vi "final drive.vi"() -> ()   [LabVIEW 2012, in "Sendmail.lvrbt"]
uses:
  Sendmail.lvrbt
  <vilib>/NXT/Block Support/NXT_MessageMailbox.ctl
  <vilib>/NXT/Hardware/Plugins/Tetrix 180 deg Servo/Tetrix180ServoAddress.ctl
  <vilib>/NXT/Hardware/Plugins/Tetrix DC Motor/TetrixDCMotorAddress.ctl
  <vilib>/NXT/Dual Mode Library/BT/BlueTooth_Read_string.vi
  <vilib>/NXT/NXTIO Xnodes/NXTIONodeSubVIs/TETRIX IO Move Servos.vi
  <vilib>/NXT/Dual Mode Library/Display/drawNumber_float.vi
  <vilib>/NXT/Dual Mode Library/Display/drawText.vi
  <vilib>/NXT/NXTIO Xnodes/NXTIONodeSubVIs/TETRIX IO Move DC Motors.vi
  <vilib>/NXT/Subs/LVHSConnector.ctl
  <vilib>/NXT/NXTIO Xnodes/AddressXNode/NXTIOAddress.xnode
  <vilib>/NXT/NXTIO Xnodes/NXTIOXNode/NXTIO.xnode
  <vilib>/NXT/LegoClasses/BrickReference/BrickReference.lvclass
panel:
  in  "String":string
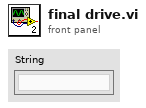
[diagram p1: front panel]
types:
  T1 = typedef "TetrixDCMotorAddress.ctl" = i16
  T2 = cluster{"TetrixDCMotor":T1, "TetrixDCMotor 2":T1}
  T3 = typedef "Tetrix180ServoAddress.ctl" = i16
  T4 = cluster{"Tetrix180Servo":T3, "Tetrix180Servo 2":T3}
  T5 = typedef "NXT_MessageMailbox.ctl" = u8
  T6 = cluster{"Tetrix180Servo":T3, "Tetrix180Servo":T3}
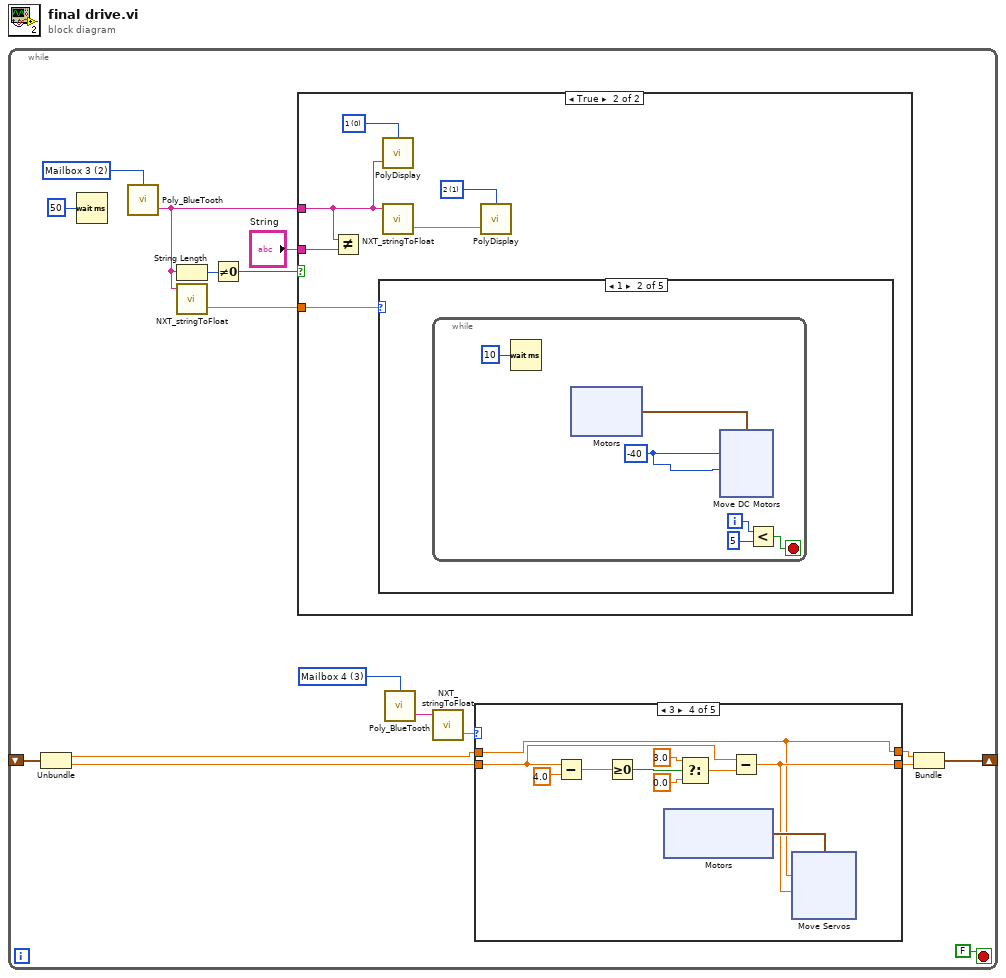
[diagram p0: block diagram]
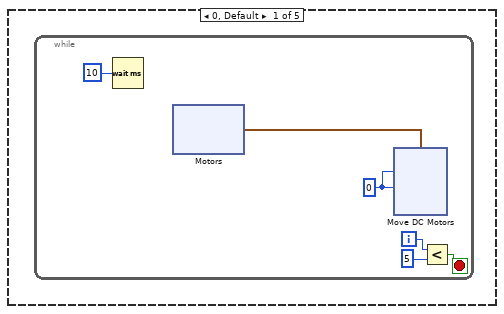
[diagram p3: hidden frame]
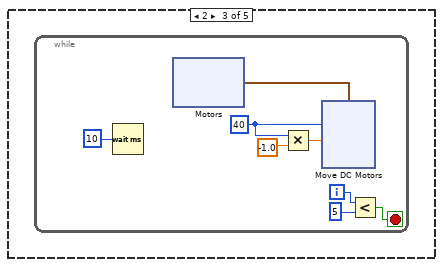
[diagram p4: hidden frame]
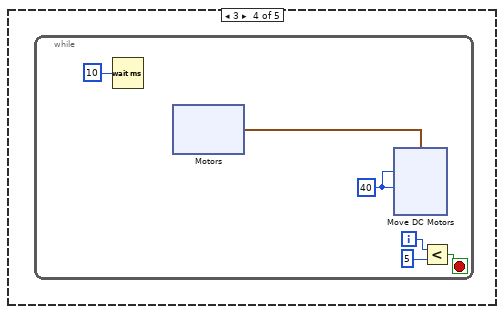
[diagram p5: hidden frame]
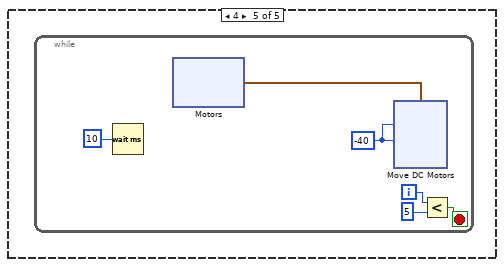
[diagram p6: hidden frame]
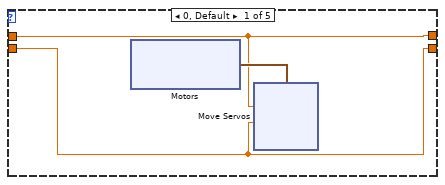
[diagram p7: hidden frame]
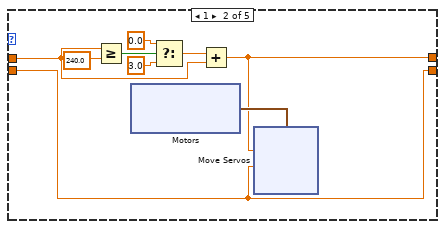
[diagram p8: hidden frame]
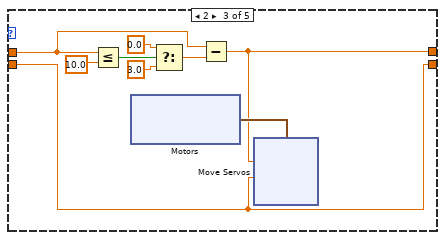
[diagram p9: hidden frame]
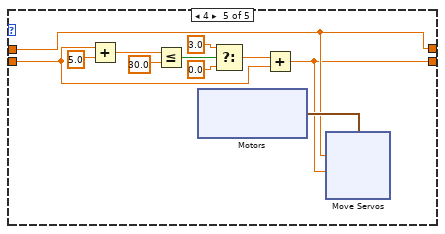
[diagram p10: hidden frame]
diagram:
  n1 = while {
    shift-right: [w12] -> _
    shift-left: _ -> [w11]
    stop <- FALSE stop-if-true
    w5 = T5 2 items=["Mailbox 1", "Mailbox 2", "Mailbox 3", "Mailbox 4", "Mailbox 5", "Mailbox 6", "Mailbox 7", "Mailbox 8", "Mailbox 9", "Mailbox 10"] ("Mailbox")
    w17 = T5 3 items=["Mailbox 1", "Mailbox 2", "Mailbox 3", "Mailbox 4", "Mailbox 5", "Mailbox 6", "Mailbox 7", "Mailbox 8", "Mailbox 9", "Mailbox 10"] ("Mailbox")
    n2 = Unbundle(w11) -> (w10:dbl, w9:dbl)
    n3 = Wait (ms)(milliseconds to wait=u32 50) -> ()  [unwired: 1 out]
    n4 = call-poly <vilib>:"Poly_BlueTooth.vi"("Mailbox"=w5) -> ("Message"=w2:string)  [unwired: 2 in, 1 out]
    n5 = String Length(string=w2) -> (length=w3:i32)
    n6 = call <vilib>:"NXT_stringToFloat.vi"("string"=w2) -> ("number"=w1:sgl)  [unwired: 2 in, 1 out]
    n7 = Not Equal To 0?(x=w3) -> (x != 0?=w6:bool)
    n8 = case shown="True" w6 {
      tunnel: w2 -> [_ w22]
      tunnel: "String" -> [_ w23]
      tunnel: w1 -> [_ w18]
      frame False {
      }
      frame True {
        w20 = i16 1 items=["1", "2", "3", "4", "5", "6", "7", "8"] ("Line")
        w21 = i16 0 items=["1", "2", "3", "4", "5", "6", "7", "8"] ("Line")
        n9 = Not Equal?(x=w22, y=w23) -> ()  [unwired: 1 out]
        n10 = case shown="1" w18 {
          frame 0, Default {
            n11 = while {
              i -> [w28]
              stop <- w25 stop-if-true
              w24 = 0 ("y")
              n12 = Wait (ms)(milliseconds to wait=u32 10) -> ()  [unwired: 1 out]
              n13 = xnode "Motors"() -> ("Motor"=w29:cluster{"TetrixDCMotor":T1, "TetrixDCMotor":T1})
              n14 = xnode "Move DC Motors"("Power/Speed 2"=w24, "Power/Speed 1"=w24, "Motors"=w29) -> ()  [unwired: 1 in, 1 out]
              n15 = Less?(x=w28, y=5) -> (x < y?=w25:bool)
            }
          }
          frame 1 {
            n16 = while {
              i -> [w45]
              stop <- w42 stop-if-true
              w41 = -40 ("y")
              n17 = Wait (ms)(milliseconds to wait=u32 10) -> ()  [unwired: 1 out]
              n18 = xnode "Motors"() -> ("Motor"=w46:cluster{"TetrixDCMotor":T1, "TetrixDCMotor":T1})
              n19 = xnode "Move DC Motors"("Power/Speed 2"=w41, "Power/Speed 1"=w41, "Motors"=w46) -> ()  [unwired: 1 in, 1 out]
              n20 = Less?(x=w45, y=5) -> (x < y?=w42:bool)
            }
          }
          frame 2 {
            n21 = while {
              i -> [w64]
              stop <- w61 stop-if-true
              w59 = 40 ("y")
              n22 = Wait (ms)(milliseconds to wait=u32 10) -> ()  [unwired: 1 out]
              n23 = xnode "Motors"() -> ("Motor"=w65:cluster{"TetrixDCMotor":T1, "TetrixDCMotor":T1})
              n24 = Multiply(x=w59, y=-1.0) -> (x*y=w58:dbl)
              n25 = xnode "Move DC Motors"("Power/Speed 2"=w58, "Power/Speed 1"=w59, "Motors"=w65) -> ()  [unwired: 1 in, 1 out]
              n26 = Less?(x=w64, y=5) -> (x < y?=w61:bool)
            }
          }
          frame 3 {
            n27 = while {
              i -> [w81]
              stop <- w78 stop-if-true
              w77 = 40 ("y")
              n28 = Wait (ms)(milliseconds to wait=u32 10) -> ()  [unwired: 1 out]
              n29 = xnode "Motors"() -> ("Motor"=w82:cluster{"TetrixDCMotor":T1, "TetrixDCMotor":T1})
              n30 = xnode "Move DC Motors"("Power/Speed 2"=w77, "Power/Speed 1"=w77, "Motors"=w82) -> ()  [unwired: 1 in, 1 out]
              n31 = Less?(x=w81, y=5) -> (x < y?=w78:bool)
            }
          }
          frame 4 {
            n32 = while {
              i -> [w98]
              stop <- w95 stop-if-true
              w94 = -40 ("y")
              n33 = Wait (ms)(milliseconds to wait=u32 10) -> ()  [unwired: 1 out]
              n34 = xnode "Motors"() -> ("Motor"=w99:cluster{"TetrixDCMotor":T1, "TetrixDCMotor":T1})
              n35 = xnode "Move DC Motors"("Power/Speed 2"=w94, "Power/Speed 1"=w94, "Motors"=w99) -> ()  [unwired: 1 in, 1 out]
              n36 = Less?(x=w98, y=5) -> (x < y?=w95:bool)
            }
          }
        }
        n37 = call-poly <vilib>:"PolyDisplay.vi"("Text"=w22, "Line"=w21) -> ()  [unwired: 2 in, 1 out]
        n38 = call <vilib>:"NXT_stringToFloat.vi"("string"=w22) -> ("number"=w19:sgl)  [unwired: 2 in, 1 out]
        n39 = call-poly <vilib>:"PolyDisplay.vi"("number"=w19, "Line"=w20) -> ()  [unwired: 2 in, 1 out]
      }
    }
    n40 = call-poly <vilib>:"Poly_BlueTooth.vi"("Mailbox"=w17) -> ("Message"=w16:string)  [unwired: 2 in, 1 out]
    n41 = call <vilib>:"NXT_stringToFloat.vi"("string"=w16) -> ("number"=w13:sgl)  [unwired: 2 in, 1 out]
    n42 = case shown="3" w13 {
      tunnel: w10 -> [w112 w125 w145 w167 w194]
      tunnel: w9 -> [w111 w132 w152 w165 w187]
      tunnel: [w112 w128 w148 w167 w194] -> w8
      tunnel: [w111 w132 w152 w168 w186] -> w7
      frame 0, Default {
        n43 = xnode "Motors"() -> ("Motor"=w113:T6)
        n44 = xnode "Move Servos"("Position 2"=w111, "Position 1"=w112, "Servos"=w113) -> ()  [unwired: 1 in, 1 out]
      }
      frame 1 {
        n45 = Greater Or Equal?(x=w125, y=240.0) -> (x >= y?=w126:bool)
        n46 = xnode "Motors"() -> ("Motor"=w133:T6)
        n47 = Select(t=0.0, s=w126, f=3.0) -> (s? t:f=w129:dbl)
        n48 = Add(x=w129, y=w125) -> (x+y=w128:dbl)
        n49 = xnode "Move Servos"("Position 2"=w132, "Position 1"=w128, "Servos"=w133) -> ()  [unwired: 1 in, 1 out]
      }
      frame 2 {
        n50 = Less Or Equal?(x=w145, y=10.0) -> (x <= y?=w146:bool)
        n51 = xnode "Motors"() -> ("Motor"=w153:T6)
        n52 = Select(t=0.0, s=w146, f=3.0) -> (s? t:f=w149:dbl)
        n53 = Subtract(x=w145, y=w149) -> (x-y=w148:dbl)
        n54 = xnode "Move Servos"("Position 2"=w152, "Position 1"=w148, "Servos"=w153) -> ()  [unwired: 1 in, 1 out]
      }
      frame 3 {
        n55 = Subtract(x=w165, y=4.0) -> (x-y=w172:dbl)
        n56 = Greater Or Equal To 0?(x=w172) -> (x >= 0?=w171:bool)
        n57 = xnode "Motors"() -> ("Motor"=w174:T6)
        n58 = Select(t=3.0, s=w171, f=0.0) -> (s? t:f=w166:dbl)
        n59 = Subtract(x=w165, y=w166) -> (x-y=w168:dbl)
        n60 = xnode "Move Servos"("Position 2"=w168, "Position 1"=w167, "Servos"=w174) -> ()  [unwired: 1 in, 1 out]
      }
      frame 4 {
        n61 = Add(x=w187, y=5.0) -> (x+y=w193:dbl)
        n62 = Less Or Equal?(x=w193, y=30.0) -> (x <= y?=w191:bool)
        n63 = xnode "Motors"() -> ("Motor"=w196:T6)
        n64 = Select(t=3.0, s=w191, f=0.0) -> (s? t:f=w188:dbl)
        n65 = Add(x=w188, y=w187) -> (x+y=w186:dbl)
        n66 = xnode "Move Servos"("Position 2"=w186, "Position 1"=w194, "Servos"=w196) -> ()  [unwired: 1 in, 1 out]
      }
    }
    n67 = Bundle(w8, w7) -> (w12:cluster{dbl, dbl})  [unwired: 1 in]
  }
